vi "Open First Controller.vi"(7 "Enable Events (T)":bool=TRUE, 8 "Error In":errorcluster) -> (0 "Error Out":errorcluster, 2 "Event Refnum":refnum<event-registration>, 3 "Xbox One Controller":T1)   [LabVIEW 2011, in "LMH-Xbox-One-Controller.lvlib"]
uses:
  LMH-Xbox-One-Controller.lvlib
  Private/Type Defs/Xbox One Controller Ref.ctl
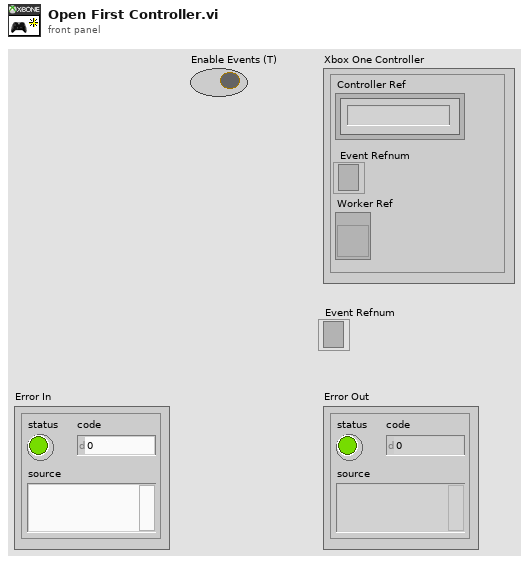
[diagram p1: front panel]
types:
  T1 = typedef "LMH-Xbox-One-Controller.lvlib/Xbox One Controller Ref.ctl" = cluster{"Controller Ref":refnum<k1>, "Event Refnum":refnum<event-registration>, "Worker Ref":refnum<vi>}
  T2 = typedef "LMH-Xbox-One-Controller.lvlib/Xbox Controller Device.ctl" = cluster{"Device Index":i32, "Device Name":string}
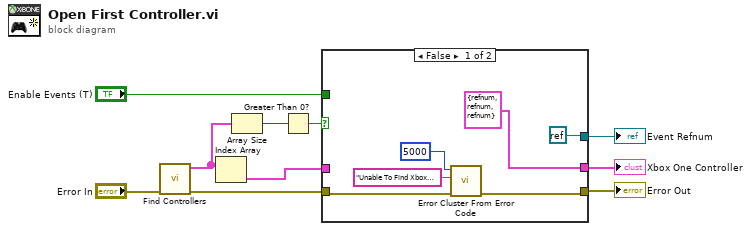
[diagram p0: block diagram]
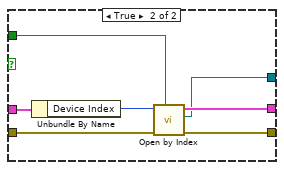
[diagram p2: hidden frame]
diagram:
  n1 = call "Find Controllers.vi"("Error In"="Error In") -> ("Error Out"=w4:errorcluster, "Xbox Controllers"=w9:T2[])  [unwired: 9 in]
  n2 = Index Array(array=w9) -> (element=w7:T2)  [unwired: 1 in]
  n3 = Array Size(array=w9) -> (size(s)=w10:i32)
  n4 = Greater Than 0?(x=w10) -> (x > 0?=w8:bool)
  n5 = case shown="False" w8 {
    tunnel: w7 -> [_ w23]
    tunnel: "Enable Events (T)" -> [_ w21]
    tunnel: w4 -> [w15 w20]
    tunnel: [w14 w19] -> w3
    tunnel: [T1 {"Controller Ref"=refnum, "Event Refnum"=refnum, "Worker Ref"=refnum} ("Xbox One Controller Ref") w18] -> w2
    tunnel: [refnum<k0> refnum w17] -> w1
    frame False {
      n6 = call <vilib>:"Error Cluster From Error Code.vi"("error in (no error)"=w15, "error message (\"\")"="Unable To Find Xbox Controller" ("error message (\"\")"), "error code (0)"=5000) -> ("error out"=w14:errorcluster)  [unwired: 6 in]
    }
    frame True {
      n7 = Unbundle By Name(w23) -> ("Device Index"=w22:i32)
      n8 = call "Open by Index.vi"("Enable Events (T)"=w21, "Error In"=w20, "Device Index"=w22) -> ("Error Out"=w19:errorcluster, "Event Refnum"=w17:refnum<event-registration>, "Xbox One Controller Ref"=w18:T1)  [unwired: 6 in]
    }
  }
  "Error Out" <- w3
  "Xbox One Controller" <- w2
  "Event Refnum" <- w1
